vi "Resize Panel to Pane.vi"(8 "error in (no error)":errorcluster, 10 "Apply Recursively? (F)":bool, 11 "IViewable In":refnum<class "IViewable.lvclass">) -> (0 "error out":errorcluster, 3 "IViewable Out":refnum<class "IViewable.lvclass">)   [LabVIEW 2015, in "IViewable.lvlib" / "IViewable.lvclass"]
doc: "<License>\nCopyright © 2017 Composed Systems, LLC | All rights reserved\nwww.composed.io\n\nAuthor: Ethan Stern <ethan.stern@composed.io>\n\nThis software is provided \"AS IS\" WITHOUT WARRANTIES, either express or implied, AND IS FOR EDUCATIONAL PURPOSES ONLY.\n</License>"
uses:
  IViewable.lvclass
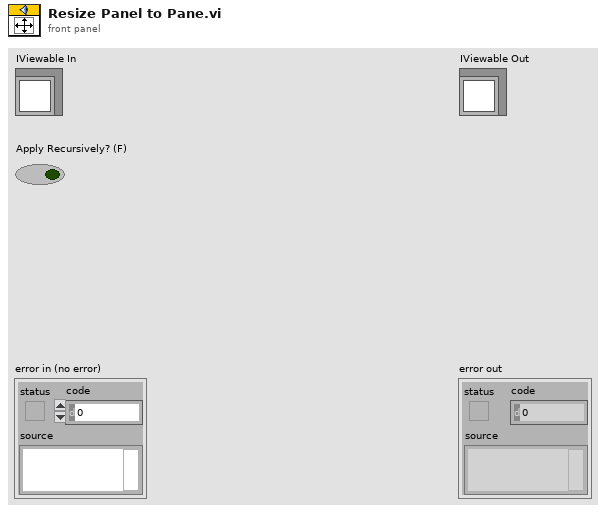
[diagram p1: front panel]
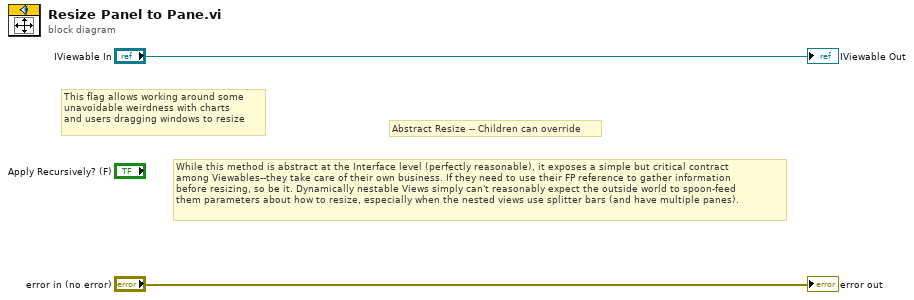
[diagram p0: block diagram]
diagram:
  # "This flag allows working around some\nunavoidable weirdness with charts\nand users dragging windows to resize"
  # "While this method is abstract at the Interface level (perfectly reasonable), it exposes a simple but critical contract\namong Viewables--they take care of their own business. If they need to use their FP reference to gather information\nbefore resizing, so be it. Dynamically nestable Views simply can't reasonably expect the outside world to spoon-feed\nthem parameters about how to resize, especially when the nested views use splitter bars (and have multiple panes)."
  # "Abstract Resize -- Children can override"
  "error out" <- "error in (no error)"
  "IViewable Out" <- "IViewable In"
